vi "Global_Spec.vi"() -> ()   [LabVIEW 2020]
panel:
  in  "Spec Temp":T1
  in  "Spec Old":T1
  in  "Spec Default":T1
  in  "Spec":T1
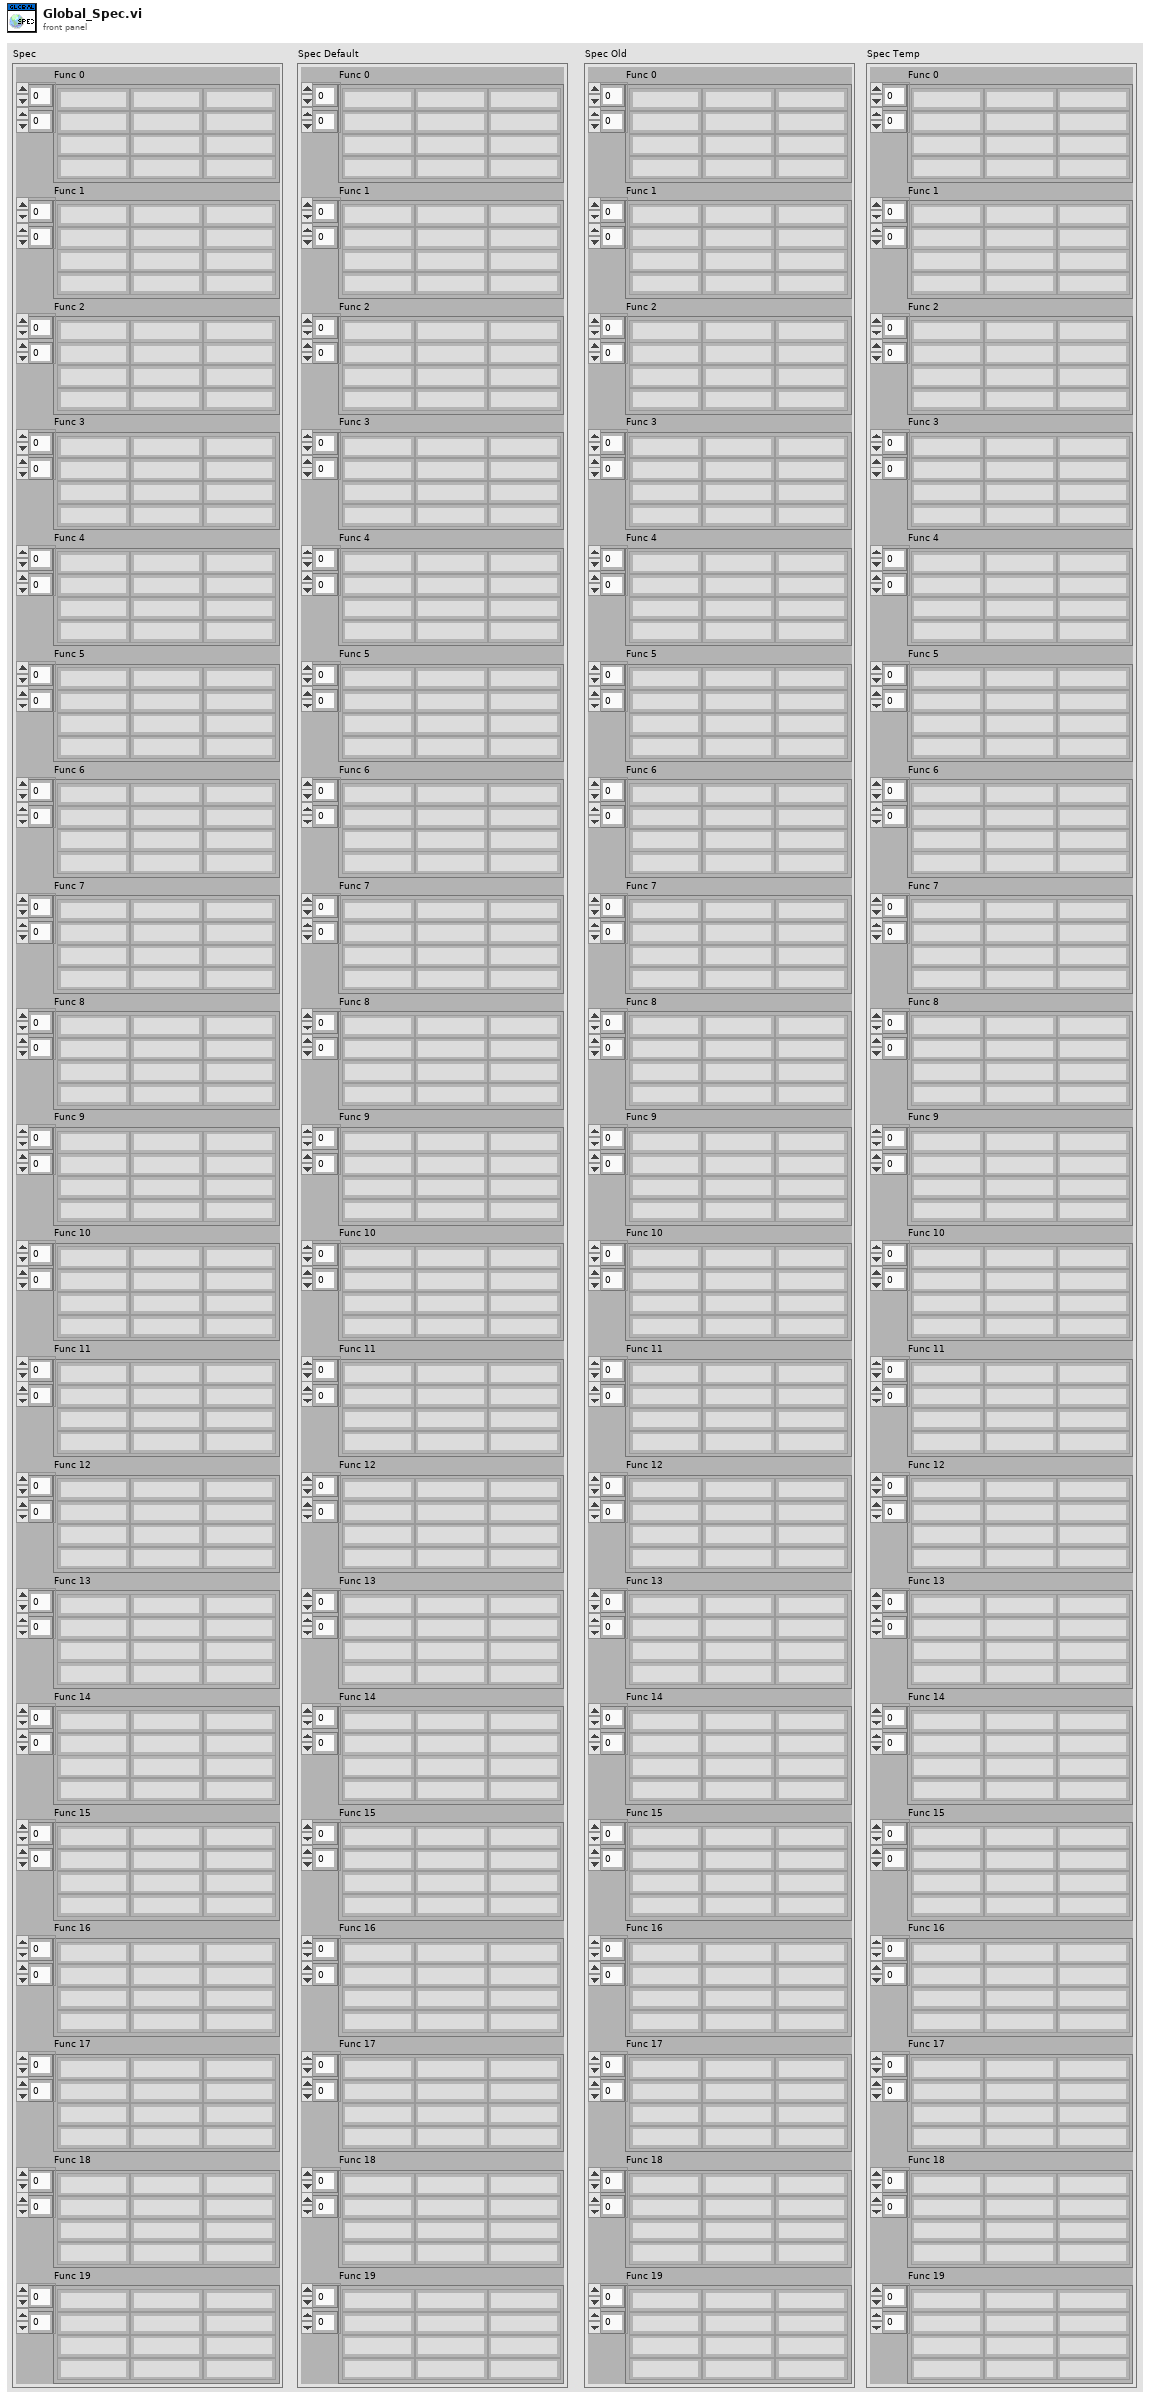
[diagram p1: front panel]
types:
  T1 = cluster{"Func 0":string[][], "Func 1":string[][], "Func 2":string[][], "Func 3":string[][], "Func 4":string[][], "Func 5":string[][], "Func 6":string[][], "Func 7":string[][], "Func 8":string[][], "Func 9":string[][], "Func 10":string[][], "Func 11":string[][], "Func 12":string[][], "Func 13":string[][], "Func 14":string[][], "Func 15":string[][], "Func 16":string[][], "Func 17":string[][], "Func 18":string[][], "Func 19":string[][]}
diagram:
